vi "Bandpass.vi"(3 "Frequency":u32, 5 "Input":fxp<+/-,24,8>) -> (1 "Output":fxp<+/-,24,8> format="%.15g")   [LabVIEW 2015]
uses:
  <vilib>/rvi/Analysis/measure/butterworth/XNode/niFpgaButterworthFilter.xnode
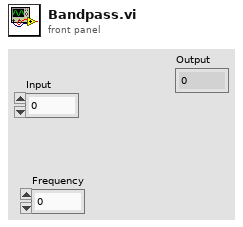
[diagram p1: front panel]
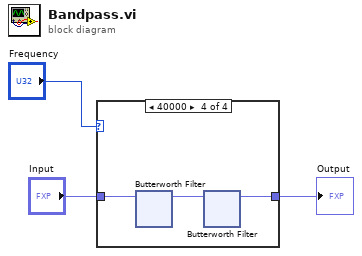
[diagram p0: block diagram]
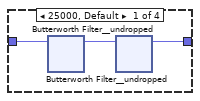
[diagram p2: hidden frame]
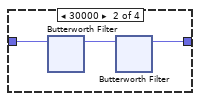
[diagram p3: hidden frame]
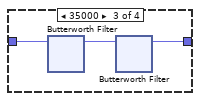
[diagram p4: hidden frame]
diagram:
  n1 = case shown="40000" "Frequency" {
    tunnel: "Input" -> [w5 w24 w43 w62]
    tunnel: [w4 w23 w42 w61] -> w1
    frame 25000, Default {
      n2 = xnode "Butterworth Filter__undropped"("input data"=w5) -> ("output data"=w6:fxp<+/-,24,8>)  [unwired: 2 in]
      n3 = xnode "Butterworth Filter__undropped"("input data"=w6) -> ("output data"=w4:fxp<+/-,24,8>)  [unwired: 2 in]
    }
    frame 30000 {
      n4 = xnode "Butterworth Filter"("input data"=w24) -> ("output data"=w25:fxp<+/-,24,8>)  [unwired: 2 in]
      n5 = xnode "Butterworth Filter"("input data"=w25) -> ("output data"=w23:fxp<+/-,24,8>)  [unwired: 2 in]
    }
    frame 35000 {
      n6 = xnode "Butterworth Filter"("input data"=w43) -> ("output data"=w44:fxp<+/-,24,8>)  [unwired: 2 in]
      n7 = xnode "Butterworth Filter"("input data"=w44) -> ("output data"=w42:fxp<+/-,24,8>)  [unwired: 2 in]
    }
    frame 40000 {
      n8 = xnode "Butterworth Filter"("input data"=w62) -> ("output data"=w63:fxp<+/-,24,8>)  [unwired: 2 in]
      n9 = xnode "Butterworth Filter"("input data"=w63) -> ("output data"=w61:fxp<+/-,24,8>)  [unwired: 2 in]
    }
  }
  "Output" <- w1
